vi "Thev-Options Dialog.vi"(0 "Cluster In":T1={"Speaker"=enum."Right primary", "Chirp"={"resol (Hz)"=50.0, "atten (dB)"=20.0, "Fs (Hz)"=100000.0}, "Find"={"precision"=10.0, "Nattempts"=6, "Navgs/att"=64}, "Gain (dB)"=40.0, "Navgs"=128, "Diameter"=0.8, "test points"=[2878.0, 3289.0, 4112.0, 4638.0, 5345.0, 7401.0], "Rprobe"=0, "LProbe"=0, "Mode"=enum."Length", "Optim"={"Fmin"=0.0, "Fmax"=0.0}} {"LProbe" items=["None"=-1, "Probe A"=0, "Probe B"=1]; "Rprobe" items=["None"=-1, "Probe A"=0, "Probe B"=1]}) -> (4 "Cluster out":T1={"Speaker"=enum."Right primary", "Chirp"={"resol (Hz)"=50.0, "atten (dB)"=20.0, "Fs (Hz)"=100000.0}, "Find"={"precision"=10.0, "Nattempts"=6, "Navgs/att"=64}, "Gain (dB)"=40.0, "Navgs"=128, "Diameter"=0.8, "test points"=[2878.0, 3289.0, 4112.0, 4638.0, 5345.0, 7401.0], "Rprobe"=0, "LProbe"=0, "Mode"=enum."Length", "Optim"={"Fmin"=0.0, "Fmax"=0.0}} {"LProbe" items=["None"=-1, "Probe A"=0, "Probe B"=1]; "Rprobe" items=["None"=-1, "Probe A"=0, "Probe B"=1]}, 8 "Canceled?":bool)   [LabVIEW 2015]
uses:
  Typedefs/Thev-Parameters.ctl
  Typedefs/Thev-Stimulus.ctl
  Typedefs/Thev-Find.ctl
  Misc VIs/Equipment Control/ER10X/ER10X-Probe.ctl
  Typedefs/Thev-Optimization Parameters.ctl
panel:
  in  "Fmax (Hz)":dbl
  in  "Fmin (Hz)":dbl
  in  "Left":i32(ring) items=["None"=-1, "Probe A"=0, "Probe B"=1]
  in  "Right":i32(ring) items=["None"=-1, "Probe A"=0, "Probe B"=1]
  out "exit signal":bool
  in  "Cancel":bool
  in  "OK":bool
  # "Probes"
  # "Optimization"
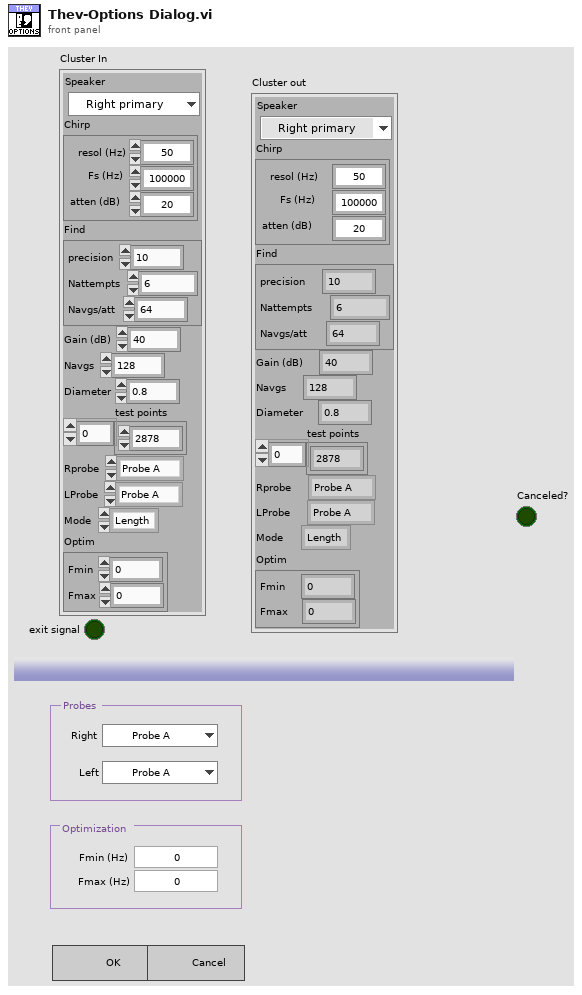
[diagram p1: front panel]
types:
  T1 = typedef "Thev-Parameters.ctl" = cluster{"Speaker":enum16{"Right primary", "Right secondary", "Left primary", "Left secondary"}, "Chirp":T2, "Find":T3, "Gain (dB)":dbl, "Navgs":i32, "Diameter":dbl, "test points":dbl[], "Rprobe":T4, "LProbe":T4, "Mode":enum16{"Length", "Freq"}, "Optim":T5}
  T2 = typedef "Thev-Stimulus.ctl" = cluster{"resol (Hz)":dbl, "atten (dB)":dbl, "Fs (Hz)":dbl}
  T3 = typedef "Thev-Find.ctl" = cluster{"precision":dbl, "Nattempts":i32, "Navgs/att":i32}
  T4 = typedef "ER10X-Probe.ctl" = i32
  T5 = typedef "Thev-Optimization Parameters.ctl" = cluster{"Fmin":dbl, "Fmax":dbl}
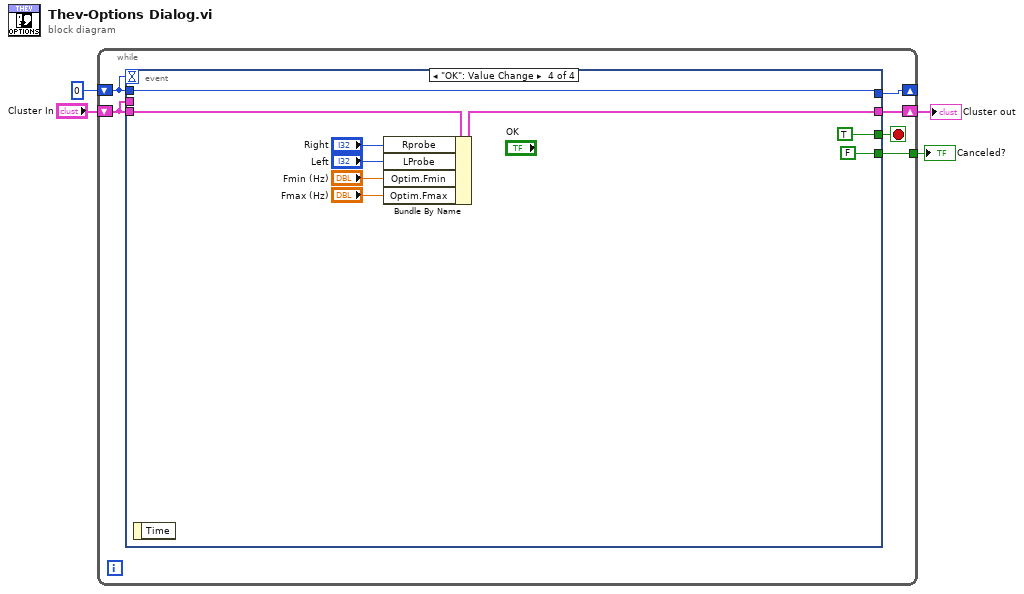
[diagram p0: block diagram]
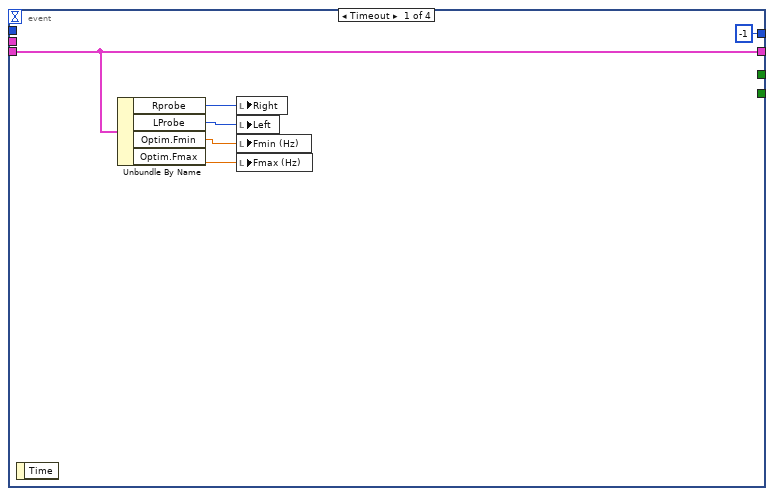
[diagram p2: hidden frame]
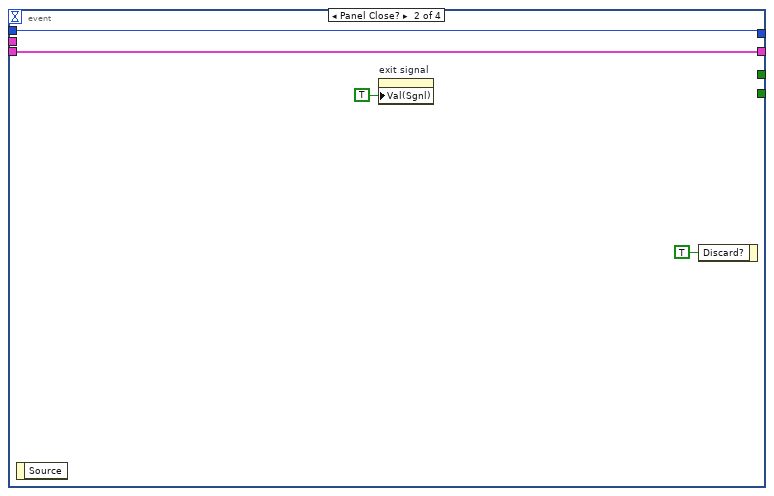
[diagram p3: hidden frame]
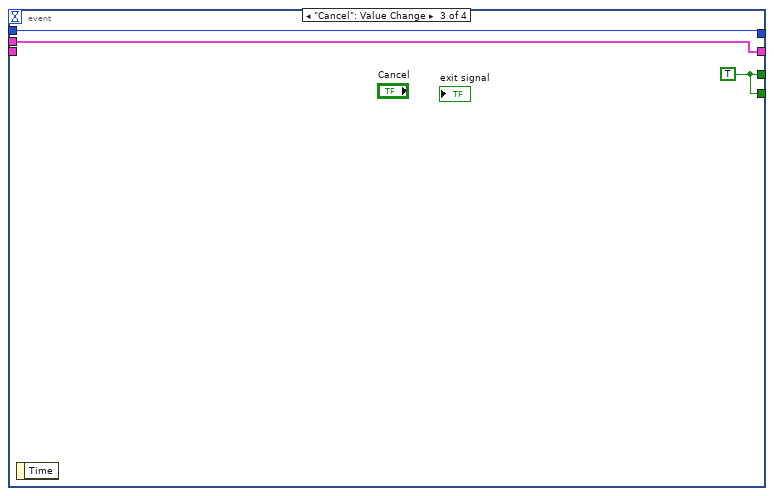
[diagram p4: hidden frame]
diagram:
  n1 = while {
    shift-right: [w10] -> _
    shift-left: 0 -> [w5]
    tunnel: [w7] -> w1
    shift-right: [w9] -> w2
    shift-left: "Cluster In" -> [w6]
    stop <- w8 stop-if-true
    n2 = event shown="[3] \"OK\": Value Change" {
      selector: _ -> [_ _ _ _]
      dyn-events: _ -> [_ _ _ _]
      timeout: w5 -> [_ _ _ _]
      tunnel: [-1 w20 w21 w29] -> w10
      tunnel: w6 -> [w15 w19 _ w32]
      tunnel: [w15 w19 w22 w28] -> w9
      tunnel: [_ _ w23 TRUE] -> w8
      tunnel: [_ _ w23 FALSE] -> w7
      tunnel: w6 -> [_ _ w22 _]
      tunnel: w5 -> [_ w20 w21 w29]
      event Timeout {
        n3 = event-data() -> ()  [unwired: 1 in, 1 out]
        n4 = Unbundle By Name(w15) -> ("Rprobe"=w14:T4, "LProbe"=w13:T4, "Optim.Fmin"=w12:dbl, "Optim.Fmax"=w11:dbl)
        n5 = local write "Right"(w14) -> ()
        n6 = local write "Left"(w13) -> ()
        n7 = local write "Fmin (Hz)"(w12) -> ()
        n8 = local write "Fmax (Hz)"(w11) -> ()
      }
      event Panel Close? {
        n9 = event-data() -> ()  [unwired: 1 in, 1 out]
        n10 = property on="exit signal" class="Bool (strict)"("Val(Sgnl)"=TRUE ("Value (Signaling)")) -> ()  [unwired: 2 in, 2 out]
        n11 = event-data("Discard?"=TRUE) -> ()  [unwired: 1 in, 1 out]
      }
      event "Cancel": Value Change {
        w23 = TRUE
        n12 = event-data() -> ()  [unwired: 1 in, 1 out]
      }
      event "OK": Value Change {
        n13 = event-data() -> ()  [unwired: 1 in, 1 out]
        n14 = Bundle By Name(cluster=w32, "Rprobe"="Right", "LProbe"="Left", "Optim.Fmin"="Fmin (Hz)", "Optim.Fmax"="Fmax (Hz)") -> (w28:T1)
      }
    }
  }
  "Cluster out" <- w2
  "Canceled?" <- w1
